vi "raw_Q_to_avg_Q.vi"(0 "scope Q data":T5, 7 "avg_Q_data":T4, 11 "Variables Cluster":T2) -> (8 "avg_Q_data out":T4, 13 "Complete Data Out":T1, 15 "error out":errorcluster)   [LabVIEW 2023]
panel:
  out "C2 Data":T3
  out "C1 Data":T3
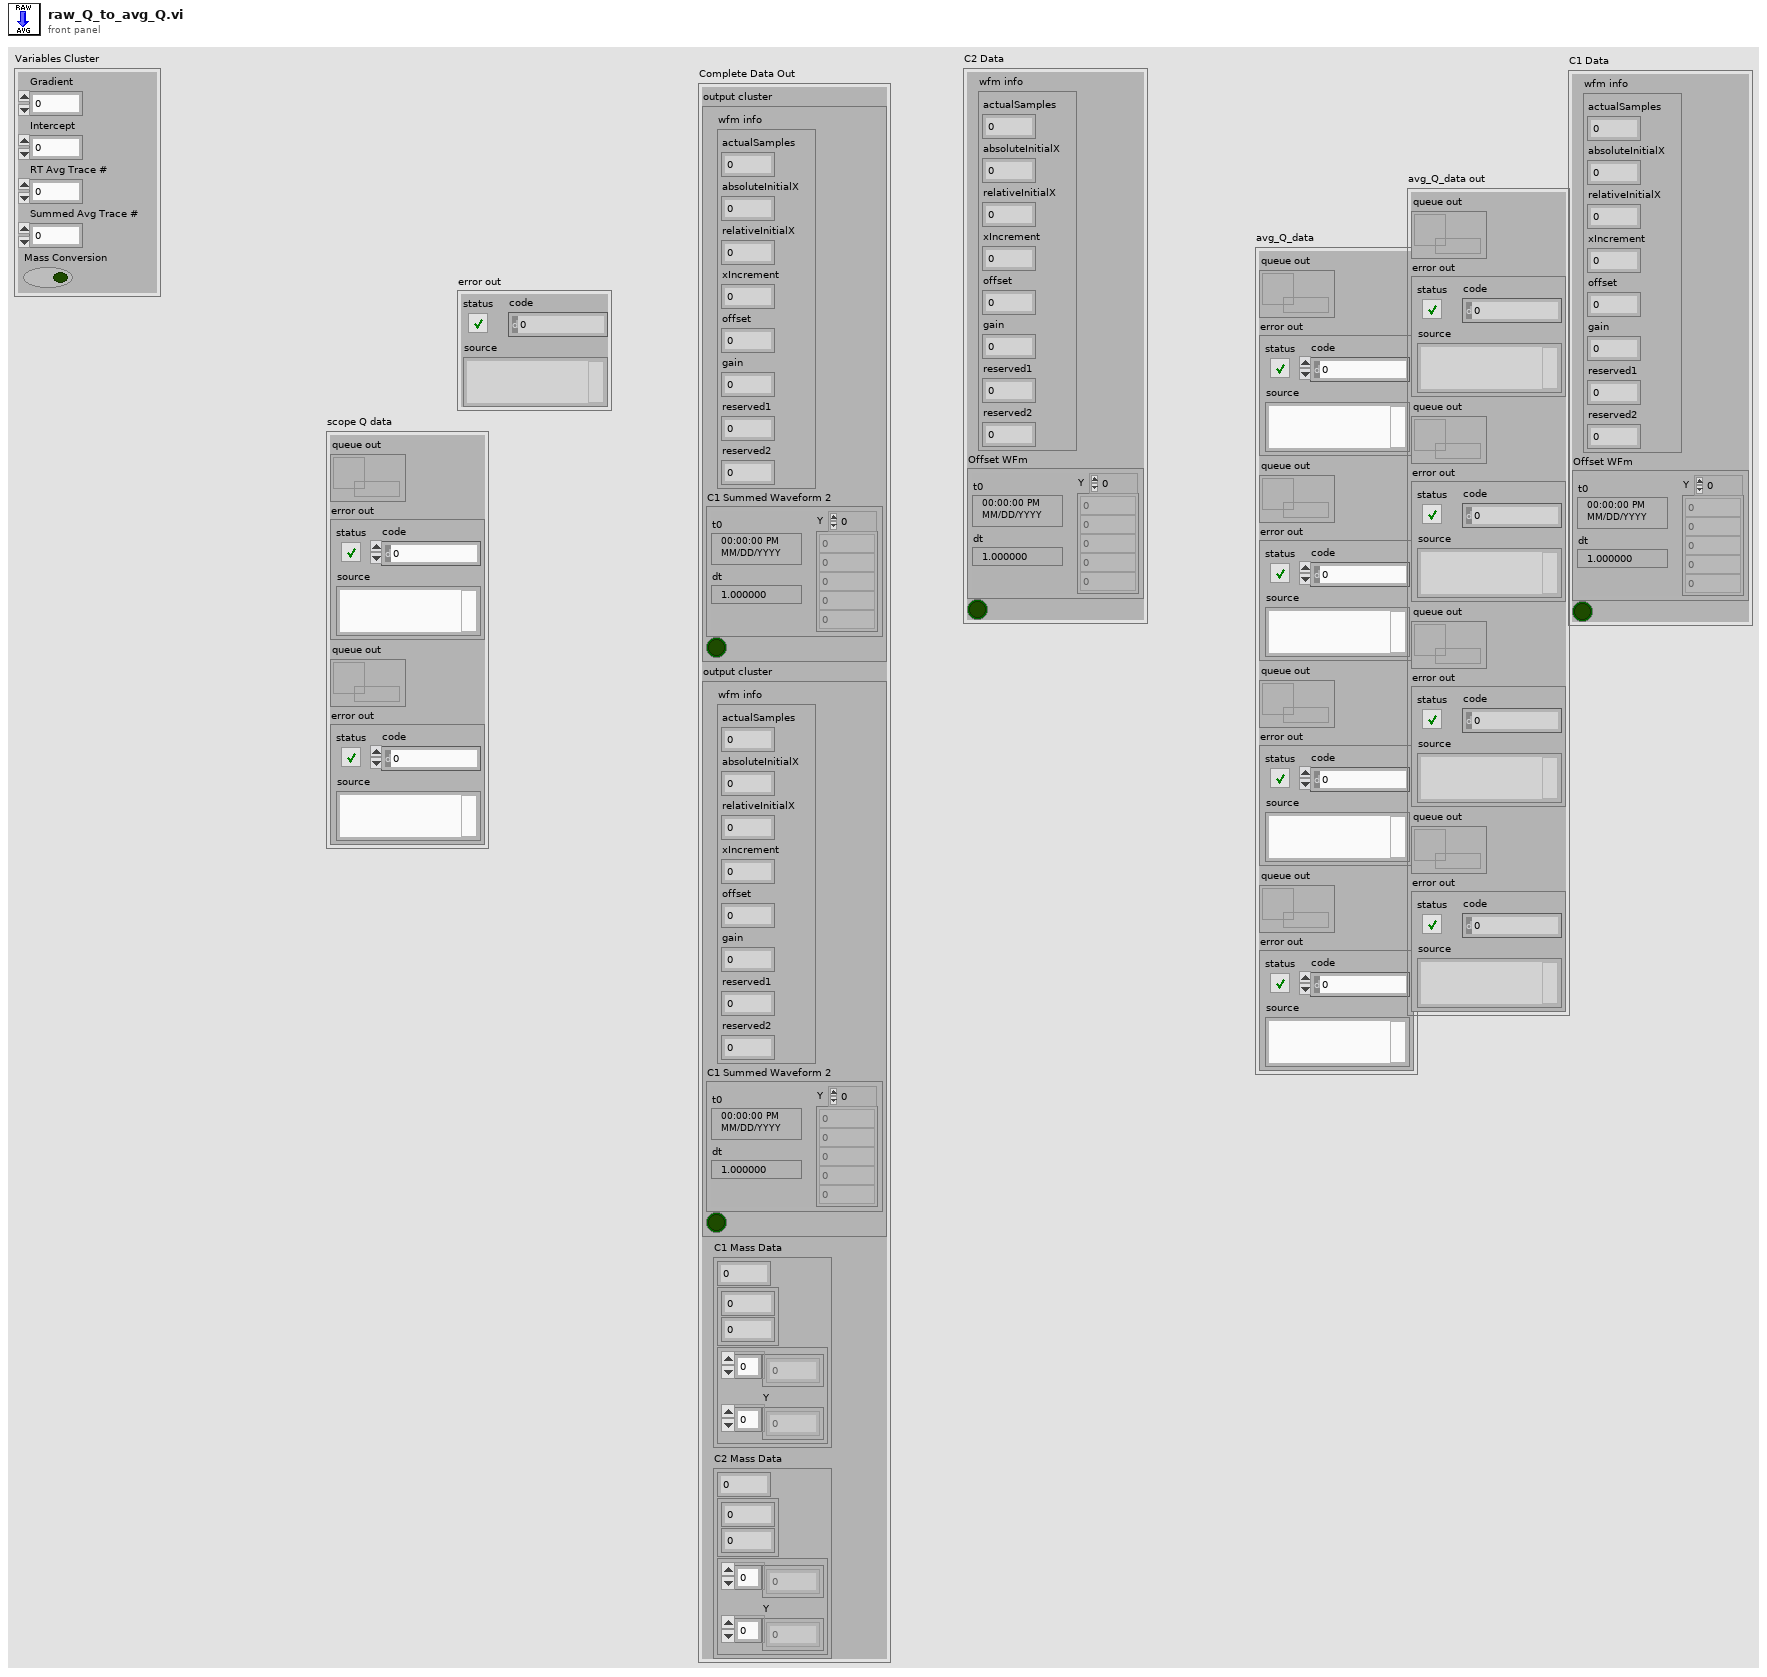
[diagram p1: front panel]
types:
  T1 = cluster{"output cluster":cluster{"wfm info":cluster{"actualSamples":i32, "absoluteInitialX":dbl, "relativeInitialX":dbl, "xIncrement":dbl, "offset":dbl, "gain":dbl, "reserved1":dbl, "reserved2":dbl}, "C1 Summed Waveform 2":waveform(dbl), bool}, "output cluster":cluster{"wfm info":cluster{"actualSamples":i32, "absoluteInitialX":dbl, "relativeInitialX":dbl, "xIncrement":dbl, "offset":dbl, "gain":dbl, "reserved1":dbl, "reserved2":dbl}, "C1 Summed Waveform 2":waveform(dbl), bool}, "C1 Mass Data":cluster{dbl, cluster{dbl, dbl}, cluster{dbl[], "Y":dbl[]}}, "C2 Mass Data":cluster{dbl, cluster{dbl, dbl}, cluster{dbl[], "Y":dbl[]}}}
  T2 = cluster{"Gradient":dbl, "Intercept":dbl, "RT Avg Trace #":i32, "Summed Avg Trace #":i32, "Mass Conversion":bool}
  T3 = cluster{"wfm info":cluster{"actualSamples":i32, "absoluteInitialX":dbl, "relativeInitialX":dbl, "xIncrement":dbl, "offset":dbl, "gain":dbl, "reserved1":dbl, "reserved2":dbl}, "Offset WFm":waveform(dbl), bool}
  T4 = cluster{"queue out":refnum<queue>, "error out":errorcluster, "queue out":refnum<queue>, "error out":errorcluster, "queue out":refnum<queue>, "error out":errorcluster, "queue out":refnum<queue>, "error out":errorcluster}
  T5 = cluster{"queue out":refnum<queue>, "error out":errorcluster, "queue out":refnum<queue>, "error out":errorcluster}
  T6 = cluster{dbl, cluster{dbl, dbl}, cluster{dbl[], "Y":dbl[]}}
  T7 = cluster{"output cluster":cluster{"wfm info":cluster{"actualSamples":i32, "absoluteInitialX":dbl, "relativeInitialX":dbl, "xIncrement":dbl, "offset":dbl, "gain":dbl, "reserved1":dbl, "reserved2":dbl}, "Offset WFm":waveform(dbl), bool}, "output cluster":cluster{"wfm info":cluster{"actualSamples":i32, "absoluteInitialX":dbl, "relativeInitialX":dbl, "xIncrement":dbl, "offset":dbl, "gain":dbl, "reserved1":dbl, "reserved2":dbl}, "Offset WFm":waveform(dbl), bool}, "C1 Mass Data":cluster{dbl, cluster{dbl, dbl}, cluster{dbl[], "Y":dbl[]}}, "C2 Mass Data":cluster{dbl, cluster{dbl, dbl}, cluster{dbl[], "Y":dbl[]}}}
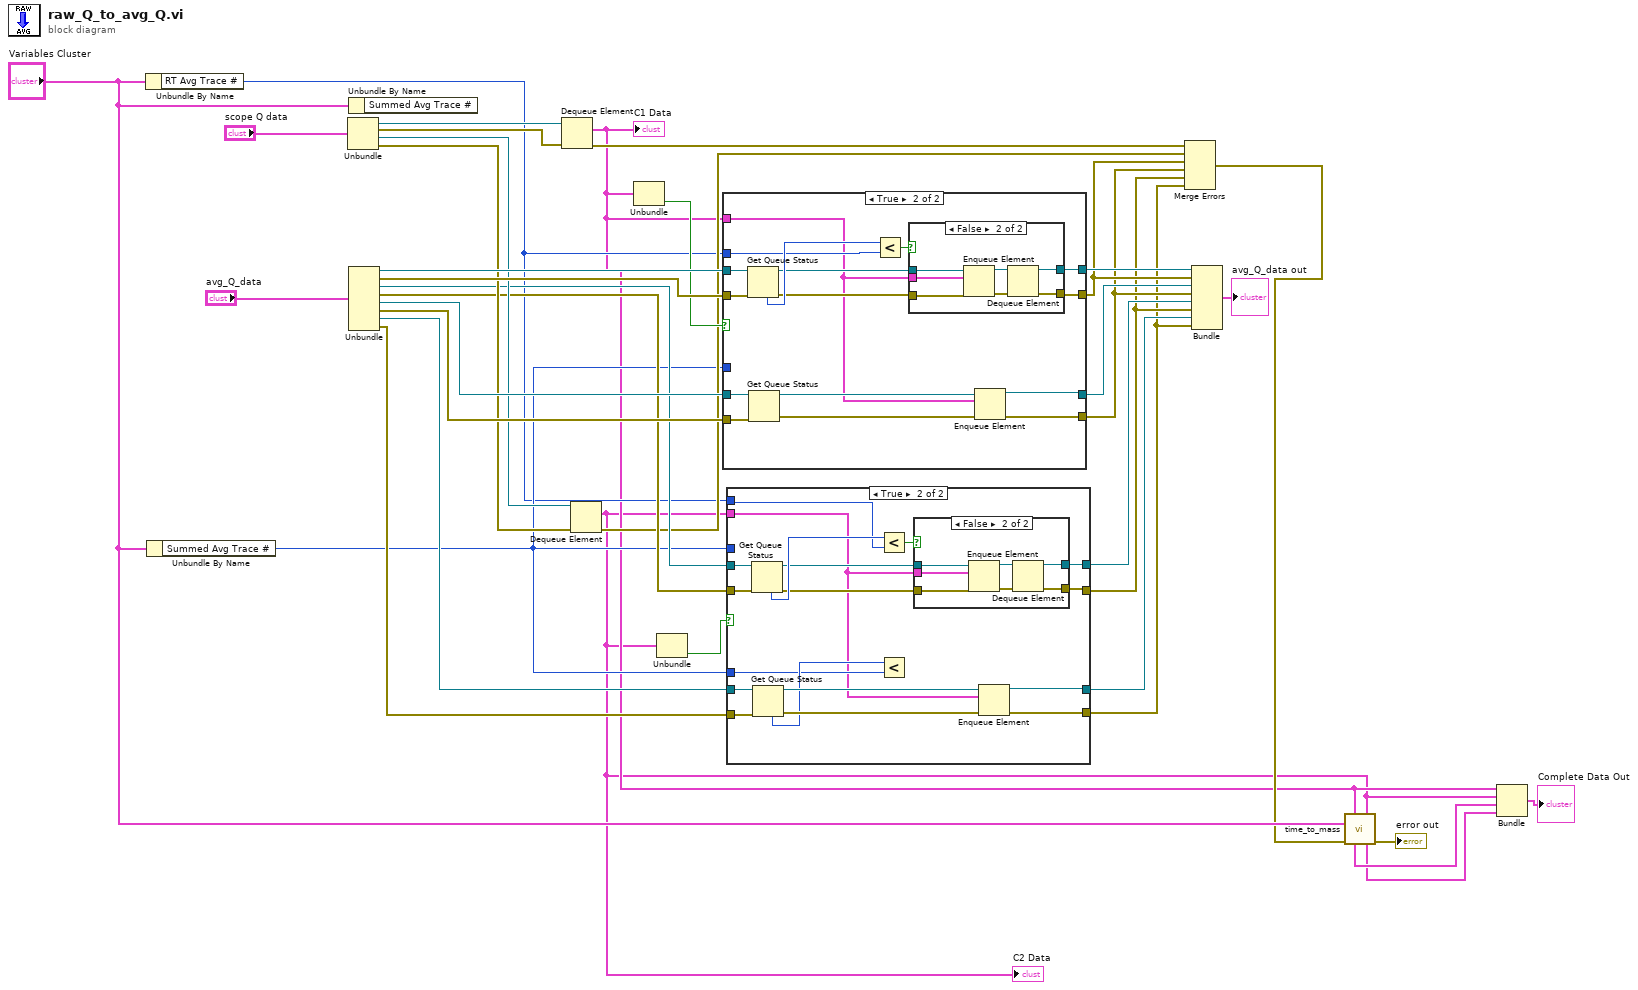
[diagram p0: block diagram]
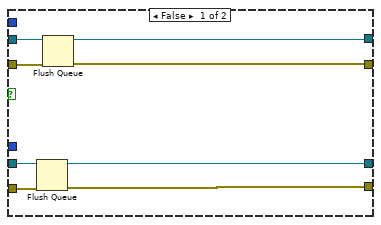
[diagram p2: hidden frame]
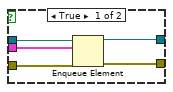
[diagram p3: hidden frame]
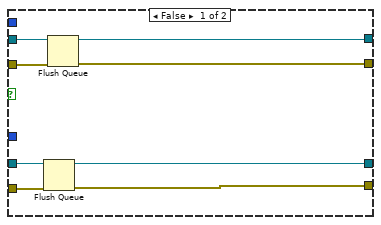
[diagram p4: hidden frame]
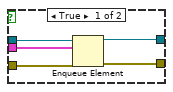
[diagram p5: hidden frame]
diagram:
  n1 = Unbundle By Name("Variables Cluster") -> ("RT Avg Trace #"=w9:i32)
  n2 = Unbundle By Name("Variables Cluster") -> ("Summed Avg Trace #"=w10:i32)
  n3 = Unbundle("scope Q data") -> ("queue out"=w35:refnum<queue>, "error out"=w34:errorcluster, "queue out"=w26:refnum<queue>, "error out"=w25:errorcluster)
  n4 = Unbundle By Name("Variables Cluster") -> ()  [unwired: 1 out]
  n5 = Unbundle("avg_Q_data") -> ("queue out"=w37:refnum<queue>, "error out"=w36:errorcluster, "queue out"=w24:refnum<queue>, "error out"=w23:errorcluster, "queue out"=w33:refnum<queue>, "error out"=w32:errorcluster, "queue out"=w22:refnum<queue>, "error out"=w21:errorcluster)
  n6 = Dequeue Element(queue=w35, error in (no error)=w34) -> (element=w5:T3, error out=w29:errorcluster)  [unwired: 1 in, 2 out]
  "C1 Data" <- w5
  n7 = Dequeue Element(queue=w26, error in (no error)=w25) -> (element=w4:T3, error out=w17:errorcluster)  [unwired: 1 in, 2 out]
  "C2 Data" <- w4
  n8 = Unbundle(w5) -> (w27:bool)  [unwired: 2 out]
  n9 = Unbundle(w4) -> (w20:bool)  [unwired: 2 out]
  n10 = case shown="True" w27 {
    tunnel: w37 -> [w45 w61]
    tunnel: w36 -> [w44 w60]
    tunnel: w33 -> [w41 w59]
    tunnel: w32 -> [w40 w58]
    tunnel: [w43 w51] -> w31
    tunnel: [w39 w57] -> w30
    tunnel: [w38 w56] -> w15
    tunnel: w5 -> [_ w47]
    tunnel: w9 -> [_ w52]
    tunnel: [w42 w50] -> w16
    tunnel: w10 -> [_ _]
    frame False {
      n11 = Flush Queue(queue=w41, error in (no error)=w40) -> (queue out=w39:refnum<queue>, error out=w38:errorcluster)  [unwired: 1 out]
      n12 = Flush Queue(queue=w45, error in (no error)=w44) -> (queue out=w43:refnum<queue>, error out=w42:errorcluster)  [unwired: 1 out]
    }
    frame True {
      n13 = Get Queue Status(queue=w61, error in (no error)=w60) -> (queue out=w49:refnum<queue>, error out=w48:errorcluster, # elements in queue=w55:i32)  [unwired: 1 in, 5 out]
      n14 = Get Queue Status(queue=w59, error in (no error)=w58) -> (queue out=w54:refnum<queue>, error out=w53:errorcluster)  [unwired: 1 in, 6 out]
      n15 = Less?(x=w55, y=w52) -> (x < y?=w46:bool)
      n16 = case shown="False" w46 {
        tunnel: w49 -> [w66 w73]
        tunnel: w48 -> [w65 w72]
        tunnel: [w64 w70] -> w51
        tunnel: [w63 w68] -> w50
        tunnel: w47 -> [w62 w67]
        frame True {
          n17 = Enqueue Element(queue=w66, element=w62, error in (no error)=w65) -> (queue out=w64:refnum<queue>, error out=w63:errorcluster)  [unwired: 1 in, 1 out]
        }
        frame False {
          n18 = Enqueue Element(queue=w73, element=w67, error in (no error)=w72) -> (queue out=w71:refnum<queue>, error out=w69:errorcluster)  [unwired: 1 in, 1 out]
          n19 = Dequeue Element(queue=w71, error in (no error)=w69) -> (queue out=w70:refnum<queue>, error out=w68:errorcluster)  [unwired: 1 in, 2 out]
        }
      }
      n20 = Enqueue Element(queue=w54, element=w47, error in (no error)=w53) -> (queue out=w57:refnum<queue>, error out=w56:errorcluster)  [unwired: 1 in, 1 out]
    }
  }
  n21 = case shown="True" w20 {
    tunnel: w24 -> [w81 w99]
    tunnel: w23 -> [w80 w98]
    tunnel: w22 -> [w77 w97]
    tunnel: w21 -> [w76 w96]
    tunnel: [w79 w87] -> w19
    tunnel: [w75 w95] -> w18
    tunnel: [w78 w86] -> w14
    tunnel: [w74 w94] -> w13
    tunnel: w4 -> [_ w83]
    tunnel: w10 -> [_ _]
    tunnel: w10 -> [_ w89]
    tunnel: w9 -> [_ w88]
    frame False {
      n22 = Flush Queue(queue=w77, error in (no error)=w76) -> (queue out=w75:refnum<queue>, error out=w74:errorcluster)  [unwired: 1 out]
      n23 = Flush Queue(queue=w81, error in (no error)=w80) -> (queue out=w79:refnum<queue>, error out=w78:errorcluster)  [unwired: 1 out]
    }
    frame True {
      n24 = Get Queue Status(queue=w99, error in (no error)=w98) -> (queue out=w85:refnum<queue>, error out=w84:errorcluster, # elements in queue=w93:i32)  [unwired: 1 in, 5 out]
      n25 = Get Queue Status(queue=w97, error in (no error)=w96) -> (queue out=w92:refnum<queue>, error out=w91:errorcluster, # elements in queue=w90:i32)  [unwired: 1 in, 5 out]
      n26 = Less?(x=w93, y=w88) -> (x < y?=w82:bool)
      n27 = Less?(x=w90, y=w89) -> ()  [unwired: 1 out]
      n28 = case shown="False" w82 {
        tunnel: w85 -> [w104 w111]
        tunnel: w84 -> [w103 w110]
        tunnel: [w102 w108] -> w87
        tunnel: [w101 w106] -> w86
        tunnel: w83 -> [w100 w105]
        frame True {
          n29 = Enqueue Element(queue=w104, element=w100, error in (no error)=w103) -> (queue out=w102:refnum<queue>, error out=w101:errorcluster)  [unwired: 1 in, 1 out]
        }
        frame False {
          n30 = Enqueue Element(queue=w111, element=w105, error in (no error)=w110) -> (queue out=w109:refnum<queue>, error out=w107:errorcluster)  [unwired: 1 in, 1 out]
          n31 = Dequeue Element(queue=w109, error in (no error)=w107) -> (queue out=w108:refnum<queue>, error out=w106:errorcluster)  [unwired: 1 in, 2 out]
        }
      }
      n32 = Enqueue Element(queue=w92, element=w83, error in (no error)=w91) -> (queue out=w95:refnum<queue>, error out=w94:errorcluster)  [unwired: 1 in, 1 out]
    }
  }
  n33 = Merge Errors(w29, w17, w16, w15, w14, w13) -> (w7:errorcluster)
  n34 = Bundle("queue out"=w31, "error out"=w16, "queue out"=w30, "error out"=w15, "queue out"=w19, "error out"=w14, "queue out"=w18, "error out"=w13) -> (→"avg_Q_data out":T4)  [unwired: 1 in]
  n35 = call "time_to_mass.vi"("C1 Data"=w5, "C2 Data"=w4, "Vairables Cluster"="Variables Cluster", "error in (no error)"=w7) -> ("C1 Mass Data"=w3:T6, "C2 Mass Data"=w2:T6, "error out"=→"error out":errorcluster)  [unwired: 9 in]
  n36 = Bundle("output cluster"=w5, "output cluster"=w4, "C1 Mass Data"=w3, "C2 Mass Data"=w2) -> (→"Complete Data Out":T7)  [unwired: 1 in]
